vi "Main.vi"() -> ()   [LabVIEW 2020]
uses:
  Test Framework/Test Framework.lvclass
panel:
  out "String (transparent)":string="WiSpry Test Framework"
  out "error IO":errorcluster
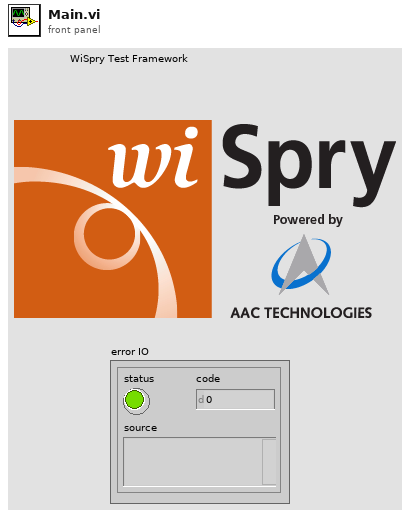
[diagram p1: front panel]
types:
  T1 = enum32{"Invalid", "Standard", "Closed", "Hidden", "Minimized", "Maximized"}
  T2 = cluster{"Restart?":bool, "User system setting file":path}
  T3 = enum32{"invalid app kind", "Development System", "Run Time System", "Student Edition", "Embedded LabVIEW", "Evaluation", "Custom"}
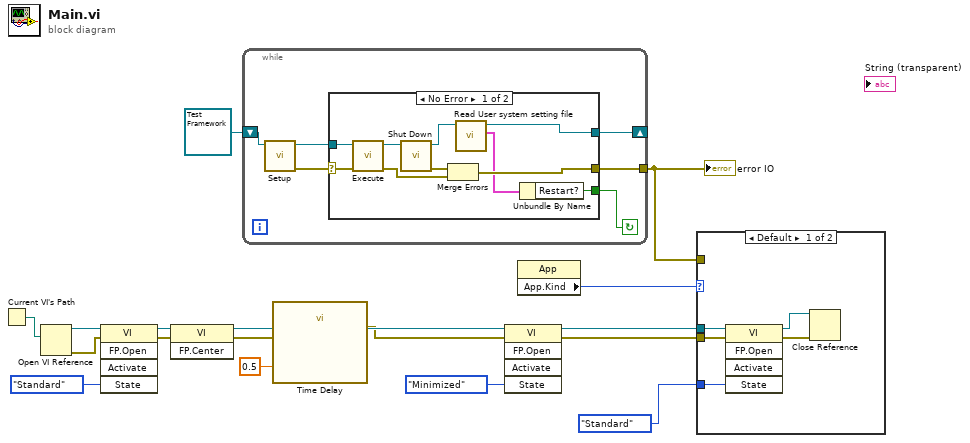
[diagram p0: block diagram]
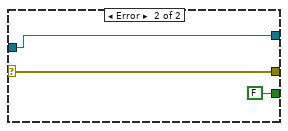
[diagram p2: hidden frame]
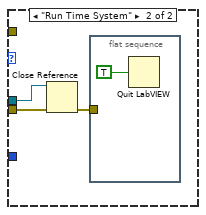
[diagram p3: hidden frame]
diagram:
  n1 = Current VI's Path() -> (path=w14:path)
  n2 = Open VI Reference(vi path=w14) -> (vi reference=w5:refnum<vi>, error out=w4:errorcluster)  [unwired: 5 in]
  n3 = invoke class="VI" method="FP.Open"(reference=w5, error in=w4, "State"=T1."Standard") -> (reference out=w8:refnum<vi>, error out=w7:errorcluster)  [unwired: 2 in, 3 out]
  n4 = invoke class="VI" method="FP.Center"(reference=w8, error in=w7) -> (reference out=w6:refnum<vi>, error out=w2:errorcluster)  [unwired: 1 in, 1 out]
  n5 = while {
    tunnel: [w21] -> w17
    shift-right: [w18] -> _
    shift-left: refnum<class "Test Framework.lvclass"> refnum ("Test Framework.lvclass") -> [w20]
    stop <- w19 continue-if-true
    n6 = call "Setup.vi"("Test Framework.lvclass"=w20) -> ("Error Out"=w22:errorcluster, "Test Framework.lvclass Out"=w23:refnum<class "Test Framework.lvclass">)  [unwired: 9 in]
    n7 = case shown="No Error" w22 {
      selector: w22 -> [w28 w36]
      tunnel: w23 -> [w33 w34]
      tunnel: [w29 w36] -> w21
      tunnel: [w25 FALSE ("Restart?")] -> w19
      tunnel: [w24 w34] -> w18
      frame No Error {
        n8 = call "Execute.vi"("Error In"=w28, "Test Framework.lvclass"=w33) -> ("Error Out"=w31:errorcluster, "Test Framework.lvclass Out"=w32:refnum<class "Test Framework.lvclass">)  [unwired: 8 in]
        n9 = call "Shut Down.vi"("Test Framework in"=w32) -> ("error out"=w30:errorcluster, "Test Framework out"=w27:refnum<class "Test Framework.lvclass">)  [unwired: 9 in]
        n10 = Merge Errors(w30, w31) -> (w29:errorcluster)
        n11 = call-dynamic "Read User system setting file.vi"("Test Framework in"=w27) -> ("User system setting file"=w26:T2, "Test Framework out"=w24:refnum<class "Test Framework.lvclass">)  [unwired: 9 in]
        n12 = Unbundle By Name(w26) -> ("Restart?"=w25:bool)
      }
      frame Error {
      }
    }
  }
  "error IO" <- w17
  n13 = call "Time Delay"("error in (no error)"=w2, "Delay Time (s)"=0.5) -> ("error out"=w1:errorcluster)  [unwired: 9 in]
  n14 = invoke class="VI" method="FP.Open"(reference=w6, error in=w1, "State"=T1."Minimized") -> (reference out=w11:refnum<vi>, error out=w10:errorcluster)  [unwired: 2 in, 3 out]
  n15 = property class="App"() -> ("App.Kind"=w15:T3)  [unwired: 2 in, 2 out]
  n16 = case shown="Default" w15 {
    tunnel: w17 -> [_ _]
    tunnel: T1."Standard" ("State") -> [w41 _]
    tunnel: w11 -> [w40 w42]
    tunnel: w10 -> [w39 w43]
    frame Default {
      n17 = invoke class="VI" method="FP.Open"(reference=w40, error in=w39, "State"=w41) -> (reference out=w37:refnum<vi>, error out=w38:errorcluster)  [unwired: 2 in, 3 out]
      n18 = Close Reference(reference=w37, error in (no error)=w38) -> ()  [unwired: 1 out]
    }
    frame "Run Time System" {
      n19 = Close Reference(reference=w42, error in (no error)=w43) -> (error out=w44:errorcluster)
      n20 = flat-sequence {
        tunnel: w44 -> [_]
        frame #0 {
          n21 = Quit LabVIEW(quit? (T)=TRUE) -> ()
        }
      }
    }
  }
